vi "dvp Vi Set Anti Flick.vi"(10 "AntiFlick":u32(ring) items=["ANTIFLICK_DISABLE", "ANTIFLICK_50HZ", "ANTIFLICK_60HZ"], 11 "handle":u32) -> (3 "function return":u32(ring))   [LabVIEW 2018, in "LabViewDVPCamera.lvlib"]
doc: "LabviewDvp2Api dvpStatus dvpViSetAntiFlick(dvpHandle handle, dvpAntiFlick AntiFlick);"
uses:
  LabViewDVPCamera.lvlib
  LabViewDVPCamera/LabViewDVPCamera.dll
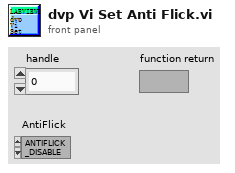
[diagram p1: front panel]
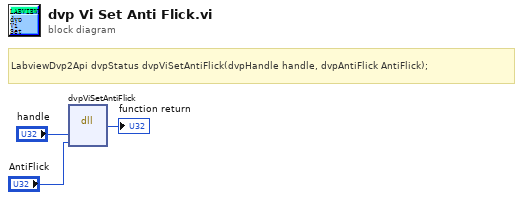
[diagram p0: block diagram]
diagram:
  # "LabviewDvp2Api dvpStatus dvpViSetAntiFlick(dvpHandle handle, dvpAntiFlick AntiFlick);"
  n1 = dll-call lib="C:/Program Files (x86)/DVP2 Labview cn 64/Sample/LabViewDVPCamera/LabViewDVPCamera.*" fn="dvpViSetAntiFlick"("handle"="handle", "AntiFlick"="AntiFlick") -> (→"function return":u32)  [unwired: 5 in, 2 out]
